vi "Periodic Tasks.vi"(8 "error in":errorcluster) -> ()   [LabVIEW 2020]
doc: "This VI runs in parallel to other tasks. It can contain as many user-defined periodic loops as you need. These can carry out PID or other sorts of timed response."
uses:
  Robot Global Data.vi
  <vilib>/Rock Robotics/Network Tables/NT Write Boolean.vi
  <vilib>/Rock Robotics/Network Tables/NT Write Numeric Array.vi
  <vilib>/Rock Robotics/Network Tables/NT Write Boolean Array.vi
  <vilib>/Rock Robotics/WPI/ThirdParty/Phoenix-LabVIEW/Motor Controller/Controls/CTRE_Phoenix_MotorControl_ControlMode.ctl
  <vilib>/Rock Robotics/WPI/RobotDrive/WPI_RobotDriveMecanumDrive_Cartesian.vi
  <vilib>/Rock Robotics/WPI/DriverStation/WPI_DriverStationRobotMode2.ctl
  <vilib>/Rock Robotics/Network Tables/NT Write Number.vi
  <vilib>/Rock Robotics/WPI/ThirdParty/Phoenix-LabVIEW/Motor Controller/Get/CTRE_Phoenix_MotorController_GetQuadratureData.vi
panel:
  out "Encoder Position":dbl
  out "Slow Speed ON":bool
  out "Backwards ON":bool
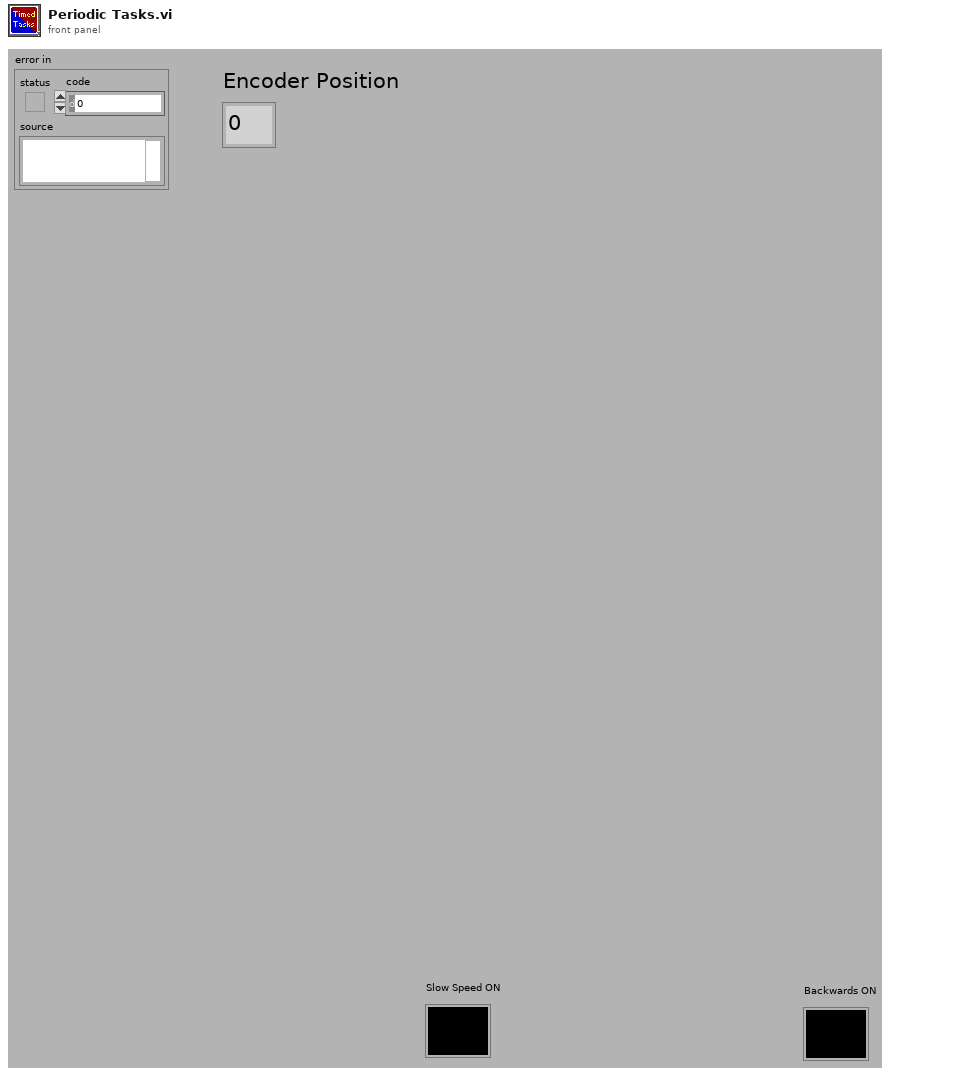
[diagram p1: front panel]
types:
  T1 = typedef "WPI_JoystickDevRef.ctl" = cluster{"Device":T2}
  T2 = typedef "WPI_JoystickDeviceEnum.ctl" = enum16{"USB 0", "USB 1", "USB 2", "USB 3", "USB 4", "USB 5"}
  T3 = typedef "WPI_RobotDriveDevRef.ctl" = cluster{"DevStatus":errorcluster, "Motors[]":T4[], "Square Inputs":bool, "Max Output":dbl}
  T4 = typedef "WPI_MotorControlDeviceRef.ctl" = cluster{"DeviceStatus":errorcluster, "Type":T5, "PWM":cluster{"PWM Channel":T6, "DeadBand":T7}, "CAN":cluster{"Device Number":u8, "SetOutput VI Ref":variant, "GetOutput VI Ref":variant, "Enable VI Ref":variant, "Disable VI Ref":variant, "Data":variant}, "Invert":bool, "DIO PWM":cluster{"PWM \"Enable\" Channel":T6, "DIOChannel":T8, "PWM Rate":dbl}}
  T5 = typedef "WPI_MotorControlType.ctl" = enum16{"PWM", "CAN", "DIO PWM"}
  T6 = typedef "FPGA_DIOPWMChannel.ctl" = enum8{"PWM 0", "PWM 1", "PWM 2", "PWM 3", "PWM 4", "PWM 5", "PWM 6", "PWM 7", "PWM 8", "PWM 9", "PWM MXP 0", "PWM MXP 1", "PWM MXP 2", "PWM MXP 3", "PWM MXP 4", "PWM MXP 5", "PWM MXP 6", "PWM MXP 7", "PWM MXP 8", "PWM MXP 9", "Invalid"}
  T7 = typedef "WPI_PWMDeadband.ctl" = cluster{"Name":string, "maxPositivePwm":i32, "minPositivePwm":i32, "centerPwm":i32, "maxNegativePwm":i32, "minNegativePwm":i32, "angularRange":u16}
  T8 = typedef "FPGA_DIOChannel.ctl" = enum8{"DIO 0", "DIO 1", "DIO 2", "DIO 3", "DIO 4", "DIO 5", "DIO 6", "DIO 7", "DIO 8", "DIO 9", "DIO MXP 0", "DIO MXP 1", "DIO MXP 2", "DIO MXP 3", "DIO MXP 4", "DIO MXP 5", "DIO MXP 6", "DIO MXP 7", "DIO MXP 8", "DIO MXP 9", "DIO MXP 10", "DIO MXP 11", "DIO MXP 12", "DIO MXP 13", "DIO MXP 14", "DIO MXP 15", "SPI Port CS1", "SPI Port CS2", "SPI Port CS3", "SPI Port MISO", "SPI Port MOSI", "Invalid"}
  T9 = typedef "WPI_ServoDeviceRef.ctl" = cluster{"DeviceStatus":errorcluster, "PWM Channel":T6, "DeadBand":T7}
  T10 = typedef "WPI_DriverStationRobotMode2.ctl" = enum16{"Autonomous Disabled", "Autonomous Enabled", "Teleop Disabled", "Teleop Enabled", "Disconnected", "Finish", "Test Disabled", "Test Enabled", "Emergency Stopped"}
  T11 = typedef "CTRE_Phoenix_MotorControl_ControlMode.ctl" = u16
  T12 = typedef "WPI_GyroDevRef.ctl" = cluster{"DevStatus":errorcluster, "Analog Channel":T13, "Gain (VoltsPerDegree/Second)":dbl, "Gyro Type":enum16{"Analog", "XRS450"}, "Handle":i32, "SPI Bus":T14, "Device Found":bool, "Sample Rate":dbl, "Calibrate On Open":bool, "Offset":dbl}
  T13 = typedef "FPGA_AIChannel.ctl" = enum8{"AI 0", "AI 1", "AI 2", "AI 3", "AI MXP 0", "AI MXP 1", "AI MXP 2", "AI MXP 3", "Invalid"}
  T14 = typedef "spi_bus.ctl" = enum16{"SPI On-Board, CS0", "SPI On-Board, CS1", "SPI On-Board, CS2", "SPI On-Board, CS3", "SPI MXP", "Invalid"}
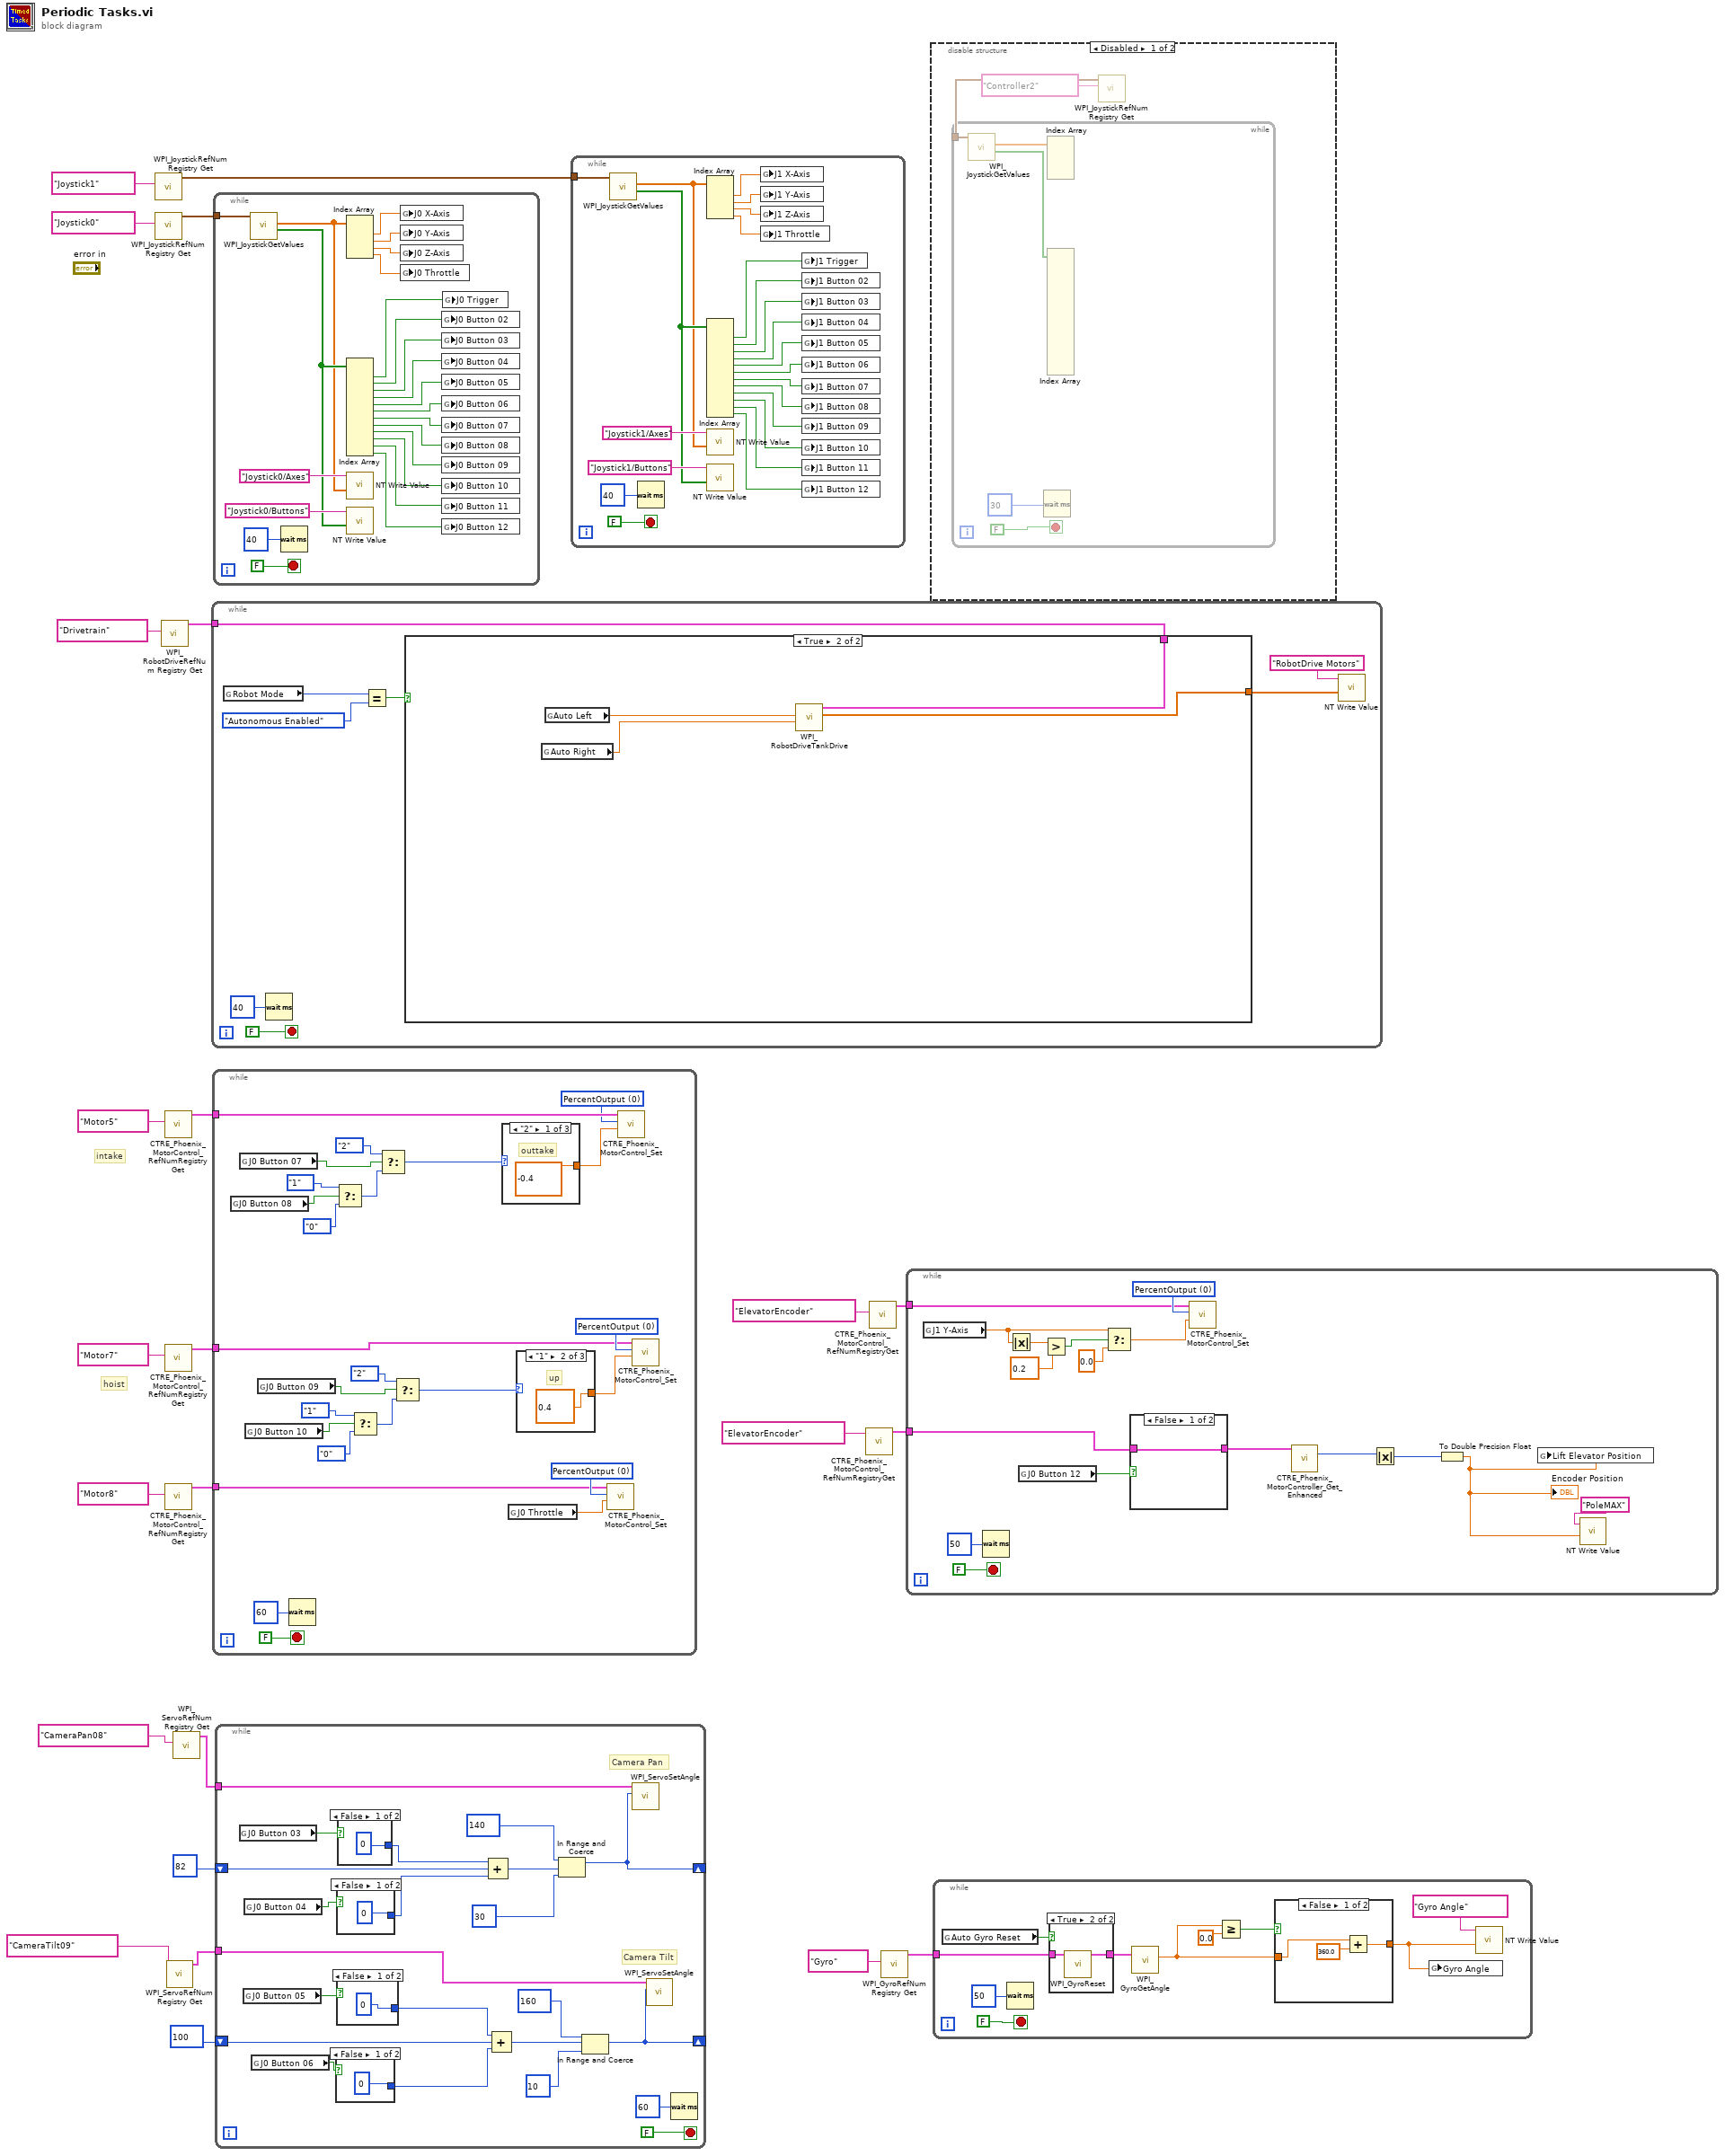
[diagram p0: block diagram]
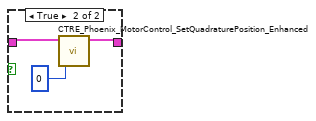
[diagram p2: hidden frame]
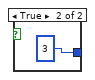
[diagram p5: hidden frame]
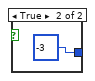
[diagram p6: hidden frame]
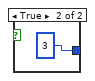
[diagram p7: hidden frame]
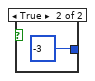
[diagram p8: hidden frame]
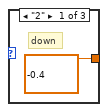
[diagram p10: hidden frame]
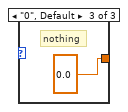
[diagram p11: hidden frame]
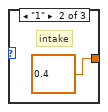
[diagram p12: hidden frame]
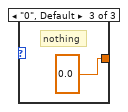
[diagram p13: hidden frame]
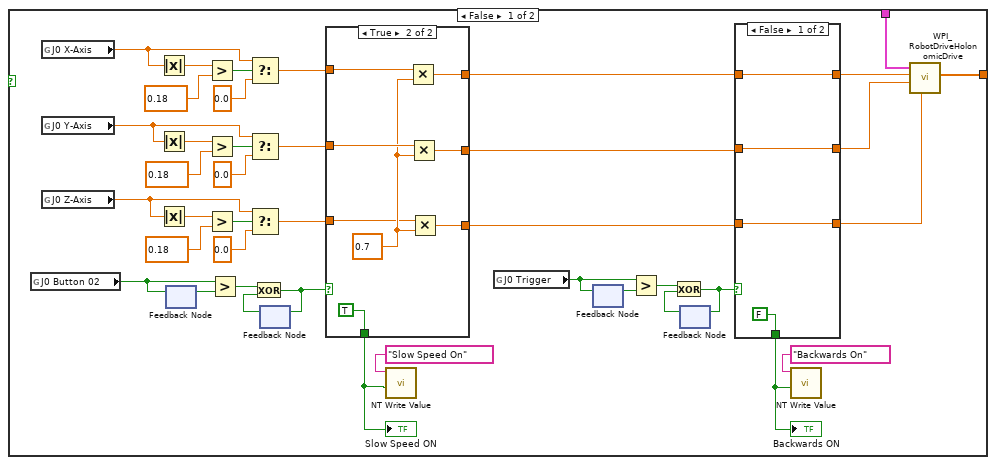
[diagram p14: hidden frame]
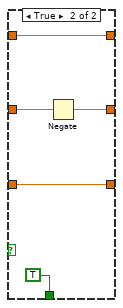
[diagram p15: hidden frame]
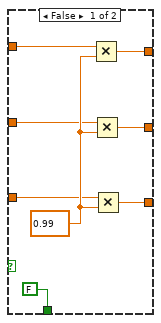
[diagram p16: hidden frame]
diagram:
  # "hoist"
  # "intake"
  n1 = call <vilib>:"WPI_JoystickRefNum Registry Get.vi"("refnum name"="Joystick1") -> ("JoystickDevRef"=w20:T1)  [unwired: 1 in, 9 out]
  n2 = call <vilib>:"WPI_JoystickRefNum Registry Get.vi"("refnum name"="Joystick0") -> ("JoystickDevRef"=w22:T1)  [unwired: 1 in, 9 out]
  n3 = call <vilib>:"WPI_RobotDriveRefNum Registry Get.vi"("refnum name"="Drivetrain") -> ("RobotDriveDevRef"=w19:T3)  [unwired: 1 in, 9 out]
  n4 = call <vilib>:"CTRE_Phoenix_MotorControl_RefNumRegistryGet.vi"("refnum name"="Motor5") -> ("PhoenixMotorControlDevRef"=w15:T4)  [unwired: 9 in, 1 out]
  n5 = call <vilib>:"CTRE_Phoenix_MotorControl_RefNumRegistryGet.vi"("refnum name"="Motor7") -> ("PhoenixMotorControlDevRef"=w14:T4)  [unwired: 9 in, 1 out]
  n6 = call <vilib>:"CTRE_Phoenix_MotorControl_RefNumRegistryGet.vi"("refnum name"="Motor8") -> ("PhoenixMotorControlDevRef"=w13:T4)  [unwired: 9 in, 1 out]
  n7 = call <vilib>:"WPI_ServoRefNum Registry Get.vi"("refnum name"="CameraTilt09") -> ("ServoDeviceRef"=w9:T9)  [unwired: 9 in, 1 out]
  n8 = call <vilib>:"WPI_ServoRefNum Registry Get.vi"("refnum name"="CameraPan08") -> ("ServoDeviceRef"=w10:T9)  [unwired: 9 in, 1 out]
  n9 = while {
    tunnel: w19 -> [w31]
    stop <- FALSE stop-if-true
    n10 = global read "Robot Global Data.vi" "Robot Mode"() -> (w27:T10)
    n11 = Wait (ms)(milliseconds to wait=u32 40) -> ()  [unwired: 1 out]
    n12 = Equal?(x=w27, y=WPI_DriverStationRobotMode2."Autonomous Enabled" ("Robot Mode")) -> (x = y?=w25:bool)
    n13 = case shown="True" w25 {
      tunnel: w31 -> [w34 w98]
      tunnel: [w33 w99] -> w30
      frame False {
        n14 = global read "Robot Global Data.vi" "J0 Button 02"() -> (w47:bool)
        n15 = global read "Robot Global Data.vi" "J0 X-Axis"() -> (w51:dbl)
        n16 = global read "Robot Global Data.vi" "J0 Y-Axis"() -> (w50:dbl)
        n17 = global read "Robot Global Data.vi" "J0 Z-Axis"() -> (w49:dbl)
        n18 = Absolute Value(x=w51) -> (abs(x)=w66:dbl)
        n19 = Absolute Value(x=w50) -> (abs(x)=w68:dbl)
        n20 = Absolute Value(x=w49) -> (abs(x)=w60:dbl)
        n21 = feedback #1() -> (w71:bool)  [unwired: 1 in]
        n22 = feedback-in #1(w47) -> ()
        n23 = Greater?(x=w66, y=0.18) -> (0:w67:bool)
        n24 = Greater?(x=w68, y=0.18) -> (0:w69:bool)
        n25 = Greater?(x=w60, y=0.18) -> (0:w61:bool)
        n26 = Greater?(x=w47, y=w71) -> (0:w70:bool)
        n27 = Select(t=w51, s=w67, f=0.0) -> (s? t:f=w52:dbl)
        n28 = Select(t=w50, s=w69, f=0.0) -> (s? t:f=w53:dbl)
        n29 = Select(t=w49, s=w61, f=0.0) -> (s? t:f=w54:dbl)
        n30 = feedback #2() -> (w72:bool)  [unwired: 1 in]
        n31 = Exclusive Or(1:w72, 2:w70) -> (0:w48:bool)
        n32 = feedback-in #2(w48) -> ()
        n33 = case shown="True" w48 {
          tunnel: w52 -> [w88 w97]
          tunnel: w53 -> [w87 w96]
          tunnel: [w85 w95] -> w40
          tunnel: [w84 w94] -> w39
          tunnel: w54 -> [w86 w92]
          tunnel: [w83 w91] -> w38
          tunnel: [FALSE ("Boolean") TRUE ("Boolean")] -> w46
          frame False {
            w89 = 0.99 ("y")
            n34 = Multiply(x=w88, y=w89) -> (x*y=w85:dbl)
            n35 = Multiply(x=w87, y=w89) -> (x*y=w84:dbl)
            n36 = Multiply(x=w86, y=w89) -> (x*y=w83:dbl)
          }
          frame True {
            w93 = 0.7 ("y")
            n37 = Multiply(x=w97, y=w93) -> (x*y=w95:dbl)
            n38 = Multiply(x=w96, y=w93) -> (x*y=w94:dbl)
            n39 = Multiply(x=w92, y=w93) -> (x*y=w91:dbl)
          }
        }
        "Slow Speed ON" <- w46
        n40 = call-poly <vilib>:"NT Write Value.vi"("Boolean"=w46, "Name"="Slow Speed On") -> ()  [unwired: 9 in, 1 out]
        n41 = global read "Robot Global Data.vi" "J0 Trigger"() -> (w45:bool)
        n42 = feedback #3() -> (w44:bool)  [unwired: 1 in]
        n43 = feedback-in #3(w45) -> ()
        n44 = Greater?(x=w45, y=w44) -> (0:w55:bool)
        n45 = feedback #4() -> (w43:bool)  [unwired: 1 in]
        n46 = Exclusive Or(1:w43, 2:w55) -> (0:w42:bool)
        n47 = feedback-in #4(w42) -> ()
        n48 = case shown="False" w42 {
          tunnel: w39 -> [w75 w80]
          tunnel: w40 -> [w73 w78]
          tunnel: [w75 w79] -> w36
          tunnel: [w73 w78] -> w35
          tunnel: w38 -> [w74 w77]
          tunnel: [w74 w77] -> w37
          tunnel: [FALSE ("Boolean") TRUE ("Boolean")] -> w41
          frame False {
          }
          frame True {
            n49 = Negate(x=w80) -> (-x=w79:dbl)
          }
        }
        "Backwards ON" <- w41
        n50 = call-poly <vilib>:"NT Write Value.vi"("Boolean"=w41, "Name"="Backwards On") -> ()  [unwired: 9 in, 1 out]
        n51 = call-poly <vilib>:"WPI_RobotDriveHolonomicDrive.vi"("Rotation"=w37, "Y"=w36, "X"=w35, "RobotDriveDevRef"=w34) -> ("Motor Values"=w33:dbl[])  [unwired: 5 in, 2 out]
      }
      frame True {
        n52 = global read "Robot Global Data.vi" "Auto Right"() -> (w100:dbl)
        n53 = global read "Robot Global Data.vi" "Auto Left"() -> (w101:dbl)
        n54 = call <vilib>:"WPI_RobotDriveTankDrive.vi"("Right axis value"=w100, "Left axis value"=w101, "RobotDriveDevRef"=w98) -> ("Motor Values"=w99:dbl[])  [unwired: 6 in, 2 out]
      }
    }
    n55 = call-poly <vilib>:"NT Write Value.vi"("Numeric Array"=w30, "Name"="RobotDrive Motors") -> ()  [unwired: 9 in, 1 out]
  }
  n56 = while {
    tunnel: w15 -> [w126]
    tunnel: w14 -> [w107]
    tunnel: w13 -> [w102]
    stop <- FALSE stop-if-true
    w104 = T11 0 items=["PercentOutput"=0, "Position"=1, "Velocity"=2, "Current"=3, "Follower"=5, "MotionProfile"=6, "MotionMagic"=7, "MotionProfileArc"=10, "Disabled"=15] ("Control Mode")
    w115 = T11 0 items=["PercentOutput"=0, "Position"=1, "Velocity"=2, "Current"=3, "Follower"=5, "MotionProfile"=6, "MotionMagic"=7, "MotionProfileArc"=10, "Disabled"=15] ("Control Mode")
    w125 = T11 0 items=["PercentOutput"=0, "Position"=1, "Velocity"=2, "Current"=3, "Follower"=5, "MotionProfile"=6, "MotionMagic"=7, "MotionProfileArc"=10, "Disabled"=15] ("Control Mode")
    n57 = global read "Robot Global Data.vi" "J0 Button 08"() -> (w105:bool)
    n58 = global read "Robot Global Data.vi" "J0 Button 07"() -> (w120:bool)
    n59 = global read "Robot Global Data.vi" "J0 Button 10"() -> (w106:bool)
    n60 = global read "Robot Global Data.vi" "J0 Button 09"() -> (w112:bool)
    n61 = Wait (ms)(milliseconds to wait=u32 60) -> ()  [unwired: 1 out]
    n62 = Select(t=enum16{"2", "1", "0", ""}."1", s=w105, f=enum16{"2", "1", "0", ""}."0") -> (s? t:f=w121:enum16{"2", "1", "0", ""})
    n63 = Select(t=enum16{"2", "1", "0", ""}."1", s=w106, f=enum16{"2", "1", "0", ""}."0") -> (s? t:f=w113:enum16{"2", "1", "0", ""})
    n64 = Select(t=enum16{"2", "1", "0", ""}."2", s=w120, f=w121) -> (s? t:f=w119:enum16{"2", "1", "0", ""})
    n65 = Select(t=enum16{"2", "1", "0", ""}."2", s=w112, f=w113) -> (s? t:f=w111:enum16{"2", "1", "0", ""})
    n66 = case shown="\"2\"" w119 {
      tunnel: [-0.4 0.4 0.0] -> w124
      frame "2" {
        # "outtake"
      }
      frame "1" {
        # "intake"
      }
      frame "0", Default {
        # "nothing"
      }
    }
    n67 = global read "Robot Global Data.vi" "J0 Throttle"() -> (w103:dbl)
    n68 = case shown="\"1\"" w111 {
      tunnel: [-0.4 0.4 0.0] -> w114
      frame "2" {
        # "down"
      }
      frame "1" {
        # "up"
      }
      frame "0", Default {
        # "nothing"
      }
    }
    n69 = call <vilib>:"CTRE_Phoenix_MotorControl_Set.vi"("Output"=w103, "Control Mode"=w104, "PhoenixMotorControlDevRef"=w102) -> ()  [unwired: 7 in, 2 out]
    n70 = call <vilib>:"CTRE_Phoenix_MotorControl_Set.vi"("Output"=w124, "Control Mode"=w125, "PhoenixMotorControlDevRef"=w126) -> ()  [unwired: 7 in, 2 out]
    n71 = call <vilib>:"CTRE_Phoenix_MotorControl_Set.vi"("Output"=w114, "Control Mode"=w115, "PhoenixMotorControlDevRef"=w107) -> ()  [unwired: 7 in, 2 out]
  }
  n72 = while {
    tunnel: w22 -> [w153]
    stop <- FALSE stop-if-true
    n73 = call <vilib>:"WPI_JoystickGetValues.vi"("JoystickDevRef"=w153) -> ("Buttons"=w134:bool[], "Axes"=w133:dbl[])  [unwired: 6 in, 3 out]
    n74 = Wait (ms)(milliseconds to wait=u32 40) -> ()  [unwired: 1 out]
    n75 = Index Array(array=w133) -> (element #1=w152:dbl, element #2=w151:dbl, element #3=w150:dbl, element #4=w149:dbl)  [unwired: 4 in]
    n76 = Index Array(array=w134) -> (element #1=w148:bool, element #2=w147:bool, element #3=w146:bool, element #4=w145:bool, element #5=w144:bool, element #6=w143:bool, element #7=w142:bool, element #8=w141:bool, element #9=w140:bool, element #10=w139:bool, element #11=w138:bool, element #12=w137:bool)  [unwired: 12 in]
    n77 = call-poly <vilib>:"NT Write Value.vi"("Numeric Array"=w133, "Name"="Joystick0/Axes") -> ()  [unwired: 9 in, 1 out]
    n78 = call-poly <vilib>:"NT Write Value.vi"("Boolean Array"=w134, "Name"="Joystick0/Buttons") -> ()  [unwired: 9 in, 1 out]
    n79 = global write "Robot Global Data.vi" "J0 X-Axis"(w152) -> ()
    n80 = global write "Robot Global Data.vi" "J0 Y-Axis"(w151) -> ()
    n81 = global write "Robot Global Data.vi" "J0 Z-Axis"(w150) -> ()
    n82 = global write "Robot Global Data.vi" "J0 Throttle"(w149) -> ()
    n83 = global write "Robot Global Data.vi" "J0 Button 02"(w147) -> ()
    n84 = global write "Robot Global Data.vi" "J0 Button 03"(w146) -> ()
    n85 = global write "Robot Global Data.vi" "J0 Button 04"(w145) -> ()
    n86 = global write "Robot Global Data.vi" "J0 Button 05"(w144) -> ()
    n87 = global write "Robot Global Data.vi" "J0 Button 06"(w143) -> ()
    n88 = global write "Robot Global Data.vi" "J0 Button 07"(w142) -> ()
    n89 = global write "Robot Global Data.vi" "J0 Button 08"(w141) -> ()
    n90 = global write "Robot Global Data.vi" "J0 Button 09"(w140) -> ()
    n91 = global write "Robot Global Data.vi" "J0 Button 10"(w139) -> ()
    n92 = global write "Robot Global Data.vi" "J0 Button 11"(w138) -> ()
    n93 = global write "Robot Global Data.vi" "J0 Button 12"(w137) -> ()
    n94 = global write "Robot Global Data.vi" "J0 Trigger"(w148) -> ()
  }
  n95 = while {
    tunnel: w10 -> [w177]
    tunnel: w9 -> [w176]
    shift-right: [w164] -> _
    shift-left: 82 -> [w157]
    shift-right: [w156] -> _
    shift-left: 100 -> [w173]
    stop <- FALSE stop-if-true
    # "Camera Tilt"
    # "Camera Pan"
    n96 = global read "Robot Global Data.vi" "J0 Button 03"() -> (w160:bool)
    n97 = global read "Robot Global Data.vi" "J0 Button 05"() -> (w162:bool)
    n98 = global read "Robot Global Data.vi" "J0 Button 04"() -> (w161:bool)
    n99 = global read "Robot Global Data.vi" "J0 Button 06"() -> (w163:bool)
    n100 = case shown="False" w163 {
      tunnel: [0 3] -> w172
      frame False {
      }
      frame True {
      }
    }
    n101 = case shown="False" w161 {
      tunnel: [0 3] -> w174
      frame False {
      }
      frame True {
      }
    }
    n102 = case shown="False" w162 {
      tunnel: [0 -3] -> w171
      frame False {
      }
      frame True {
      }
    }
    n103 = case shown="False" w160 {
      tunnel: [0 -3] -> w175
      frame False {
      }
      frame True {
      }
    }
    n104 = Compound Arithmetic op=ADD(w175, w157, w174) -> (w168:i32)
    n105 = Compound Arithmetic op=ADD(w171, w173, w172) -> (w165:i32)
    n106 = In Range and Coerce(upper limit=140, x=w168, lower limit=30) -> (coerced(x)=w164:i32)  [unwired: 1 out]
    n107 = In Range and Coerce(upper limit=160, x=w165, lower limit=10) -> (coerced(x)=w156:i32)  [unwired: 1 out]
    n108 = call <vilib>:"WPI_ServoSetAngle.vi"("Angle"=w164, "ServoDeviceRef"=w177) -> ()  [unwired: 8 in, 2 out]
    n109 = call <vilib>:"WPI_ServoSetAngle.vi"("Angle"=w156, "ServoDeviceRef"=w176) -> ()  [unwired: 8 in, 2 out]
    n110 = Wait (ms)(milliseconds to wait=u32 60) -> ()  [unwired: 1 out]
  }
  n111 = while {
    tunnel: w20 -> [w206]
    stop <- FALSE stop-if-true
    n112 = call <vilib>:"WPI_JoystickGetValues.vi"("JoystickDevRef"=w206) -> ("Buttons"=w187:bool[], "Axes"=w186:dbl[])  [unwired: 6 in, 3 out]
    n113 = Wait (ms)(milliseconds to wait=u32 40) -> ()  [unwired: 1 out]
    n114 = Index Array(array=w186) -> (element #1=w205:dbl, element #2=w204:dbl, element #3=w203:dbl, element #4=w202:dbl)  [unwired: 4 in]
    n115 = Index Array(array=w187) -> (element #1=w201:bool, element #2=w200:bool, element #3=w199:bool, element #4=w198:bool, element #5=w197:bool, element #6=w196:bool, element #7=w195:bool, element #8=w194:bool, element #9=w193:bool, element #10=w192:bool, element #11=w191:bool, element #12=w190:bool)  [unwired: 12 in]
    n116 = call-poly <vilib>:"NT Write Value.vi"("Numeric Array"=w186, "Name"="Joystick1/Axes") -> ()  [unwired: 9 in, 1 out]
    n117 = call-poly <vilib>:"NT Write Value.vi"("Boolean Array"=w187, "Name"="Joystick1/Buttons") -> ()  [unwired: 9 in, 1 out]
    n118 = global write "Robot Global Data.vi" "J1 X-Axis"(w205) -> ()
    n119 = global write "Robot Global Data.vi" "J1 Y-Axis"(w204) -> ()
    n120 = global write "Robot Global Data.vi" "J1 Z-Axis"(w203) -> ()
    n121 = global write "Robot Global Data.vi" "J1 Throttle"(w202) -> ()
    n122 = global write "Robot Global Data.vi" "J1 Trigger"(w201) -> ()
    n123 = global write "Robot Global Data.vi" "J1 Button 02"(w200) -> ()
    n124 = global write "Robot Global Data.vi" "J1 Button 03"(w199) -> ()
    n125 = global write "Robot Global Data.vi" "J1 Button 04"(w198) -> ()
    n126 = global write "Robot Global Data.vi" "J1 Button 05"(w197) -> ()
    n127 = global write "Robot Global Data.vi" "J1 Button 06"(w196) -> ()
    n128 = global write "Robot Global Data.vi" "J1 Button 07"(w195) -> ()
    n129 = global write "Robot Global Data.vi" "J1 Button 08"(w194) -> ()
    n130 = global write "Robot Global Data.vi" "J1 Button 09"(w193) -> ()
    n131 = global write "Robot Global Data.vi" "J1 Button 10"(w192) -> ()
    n132 = global write "Robot Global Data.vi" "J1 Button 11"(w191) -> ()
    n133 = global write "Robot Global Data.vi" "J1 Button 12"(w190) -> ()
  }
  n134 = call <vilib>:"CTRE_Phoenix_MotorControl_RefNumRegistryGet.vi"("refnum name"="ElevatorEncoder") -> ("PhoenixMotorControlDevRef"=w3:T4)  [unwired: 9 in, 1 out]
  n135 = call <vilib>:"CTRE_Phoenix_MotorControl_RefNumRegistryGet.vi"("refnum name"="ElevatorEncoder") -> ("PhoenixMotorControlDevRef"=w1:T4)  [unwired: 9 in, 1 out]
  n136 = call <vilib>:"WPI_GyroRefNum Registry Get.vi"("refnum name"="Gyro") -> ("GyroDevRef"=w7:T12)  [unwired: 9 in, 1 out]
  n137 = while {
    tunnel: w3 -> [w223]
    tunnel: w1 -> [w215]
    stop <- FALSE stop-if-true
    w216 = T11 0 items=["PercentOutput"=0, "Position"=1, "Velocity"=2, "Current"=3, "Follower"=5, "MotionProfile"=6, "MotionMagic"=7, "MotionProfileArc"=10, "Disabled"=15] ("Control Mode")
    n138 = global read "Robot Global Data.vi" "J1 Y-Axis"() -> (w212:dbl)
    n139 = Wait (ms)(milliseconds to wait=u32 50) -> ()  [unwired: 1 out]
    n140 = Absolute Value(x=w212) -> (abs(x)=w214:dbl)
    n141 = global read "Robot Global Data.vi" "J0 Button 12"() -> (w222:bool)
    n142 = Greater?(x=w214, y=0.2) -> (0:w211:bool)
    n143 = Select(t=w212, s=w211, f=0.0) -> (s? t:f=w209:dbl)
    n144 = case shown="False" w222 {
      tunnel: [w226 w228] -> w221
      tunnel: w223 -> [w226 w227]
      frame False {
      }
      frame True {
        n145 = call <vilib>:"CTRE_Phoenix_MotorControl_SetQuadraturePosition_Enhanced.vi"("New Position"=0, "PhoenixMotorControlDevRef"=w227) -> ("PhoenixMotorControlDevRef"=w228:T4)  [unwired: 8 in, 1 out]
      }
    }
    n146 = call <vilib>:"CTRE_Phoenix_MotorControl_Set.vi"("Output"=w209, "Control Mode"=w216, "PhoenixMotorControlDevRef"=w215) -> ()  [unwired: 7 in, 2 out]
    n147 = call-poly <vilib>:"CTRE_Phoenix_MotorController_Get_Enhanced.vi"("PhoenixMotorControlDevRef"=w221) -> ("Quadrature Position"=w220:i32)  [unwired: 11 in, 3 out]
    n148 = Absolute Value(x=w220) -> (abs(x)=w219:i32)
    n149 = To Double Precision Float(number=w219) -> (double precision float=w217:dbl)
    "Encoder Position" <- w217
    n150 = global write "Robot Global Data.vi" "Lift Elevator Position"(w217) -> ()
    n151 = call-poly <vilib>:"NT Write Value.vi"("Numeric"=w217, "Name"="PoleMAX") -> ()  [unwired: 9 in, 1 out]
  }
  n152 = disable-structure shown="Disabled" {
    frame Disabled {
      n153 = call <vilib>:"WPI_JoystickRefNum Registry Get.vi"("refnum name"="Controller2") -> ("JoystickDevRef"=w230:T1)  [unwired: 1 in, 9 out]
      n154 = while {
        tunnel: w230 -> [w236]
        stop <- FALSE stop-if-true
        n155 = call <vilib>:"WPI_JoystickGetValues.vi"("JoystickDevRef"=w236) -> ("Buttons"=w232:bool[], "Axes"=w233:dbl[])  [unwired: 6 in, 3 out]
        n156 = Wait (ms)(milliseconds to wait=u32 30) -> ()  [unwired: 1 out]
        n157 = Index Array(array=w233) -> ()  [unwired: 4 in, 4 out]
        n158 = Index Array(array=w232) -> ()  [unwired: 16 in, 16 out]
      }
    }
    frame Enabled {
    }
  }
  n159 = while {
    tunnel: w7 -> [w246]
    stop <- FALSE stop-if-true
    n160 = global read "Robot Global Data.vi" "Auto Gyro Reset"() -> (w244:bool)
    n161 = Wait (ms)(milliseconds to wait=u32 50) -> ()  [unwired: 1 out]
    n162 = case shown="True" w244 {
      tunnel: w246 -> [w251 w253]
      tunnel: [w251 w252] -> w245
      frame False {
      }
      frame True {
        n163 = call <vilib>:"WPI_GyroReset.vi"("GyroDevRef"=w253) -> ("GyroDevRef"=w252:T12)  [unwired: 9 in, 1 out]
      }
    }
    n164 = call <vilib>:"WPI_GyroGetAngle.vi"("GyroDevRef"=w245) -> ("Angle"=w241:dbl)  [unwired: 6 in, 4 out]
    n165 = Greater Or Equal?(x=w241, y=0.0) -> (x >= y?=w239:bool)
    n166 = case shown="False" w239 {
      tunnel: w241 -> [w248 w250]
      tunnel: [w247 w250] -> w237
      frame False {
        n167 = Add(x=w248, y=360.0) -> (x+y=w247:dbl)
      }
      frame True {
      }
    }
    n168 = global write "Robot Global Data.vi" "Gyro Angle"(w237) -> ()
    n169 = call-poly <vilib>:"NT Write Value.vi"("Numeric"=w237, "Name"="Gyro Angle" ("refnum name")) -> ()  [unwired: 9 in, 1 out]
  }
